vi "Initialize-object.vi"(7 "Main VI ref":refnum<vi>, 8 "error in (no error)":errorcluster, 9 "Client channel":refnum<queue>, 10 "Server channel":refnum<queue>) -> (0 "error out":errorcluster, 3 "Object ref out":T1)   [LabVIEW 2013, in "SLMControl.lvlib" / "SC-Main.lvclass"]
uses:
  SC-Main.lvclass
  Object-reference.ctl
  SA-SLMAPI/Sources/Message.lvclass
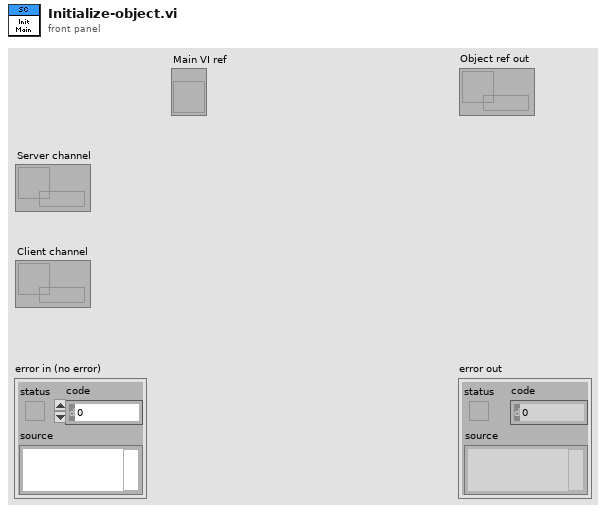
[diagram p1: front panel]
types:
  T1 = typedef "SLMControl.lvlib/SC-Main.lvclass/Object-reference.ctl" = refnum<data-value>
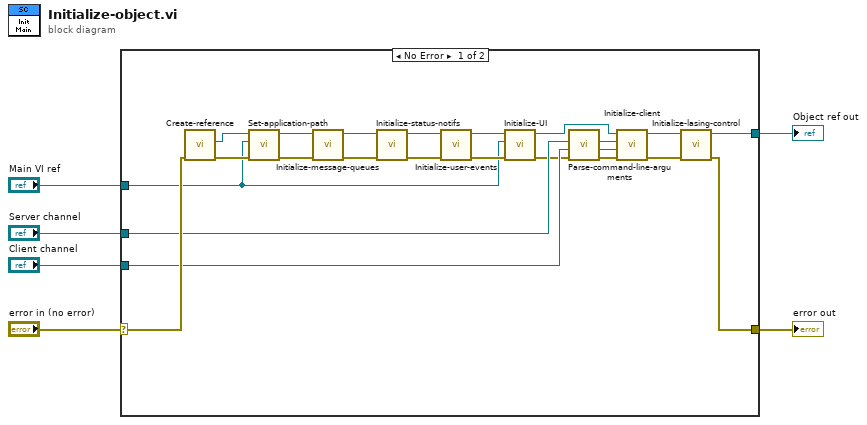
[diagram p0: block diagram]
diagram:
  n1 = case shown="No Error" "error in (no error)" {
    selector: "error in (no error)" -> [w22 w30]
    tunnel: [w18 w30] -> w5
    tunnel: [w19 _] -> w4
    tunnel: "Main VI ref" -> [w13 _]
    tunnel: "Server channel" -> [w12 _]
    tunnel: "Client channel" -> [w11 _]
    frame No Error {
      n2 = call "Create-reference.vi"("error in (no error)"=w22) -> ("error out"=w17:errorcluster, "Data ref"=w14:T1)  [unwired: 8 in, 1 out]
      n3 = call "Set-application-path.vi"("error in (no error)"=w17, "Main VI ref"=w13, "Data ref. in"=w14) -> ("error out"=w15:errorcluster, "Data ref."=w16:T1)  [unwired: 7 in]
      n4 = call "Initialize-message-queues.vi"("error in (no error)"=w15, "Object ref in"=w16) -> ("error out"=w25:errorcluster, "Object ref out"=w29:T1)  [unwired: 8 in]
      n5 = call "Initialize-status-notifs.vi"("error in (no error)"=w25, "Object ref in"=w29) -> ("error out"=w24:errorcluster, "Object ref out"=w28:T1)  [unwired: 8 in]
      n6 = call "Initialize-user-events.vi"("error in (no error)"=w24, "Object ref in"=w28) -> ("error out"=w23:errorcluster, "Object ref out"=w27:T1)  [unwired: 8 in]
      n7 = call "Initialize-UI.vi"("error in (no error)"=w23, "Main VI ref"=w13, "Object ref in"=w27) -> ("error out"=w10:errorcluster, "Object ref out"=w26:T1)  [unwired: 7 in]
      n8 = call "Parse-command-line-arguments.vi"("error in (no error)"=w10, "Client channel in"=w11, "Server channel in"=w12) -> ("error out"=w9:errorcluster, "Client channel"=w8:refnum<queue>, "Server channel"=w7:refnum<queue>)  [unwired: 6 in]
      n9 = call "Initialize-client.vi"("error in (no error)"=w9, "Client channel"=w8, "Server channel"=w7, "Object ref in"=w26) -> ("error out"=w20:errorcluster, "Object ref out"=w21:T1)  [unwired: 6 in]
      n10 = call "Initialize-lasing-control.vi"("error in (no error)"=w20, "TP-Data in"=w21) -> ("error out"=w18:errorcluster, "TP-Data out"=w19:T1)  [unwired: 8 in]
    }
    frame Error {
    }
  }
  "error out" <- w5
  "Object ref out" <- w4
